vi "Stop Log and Sequence.vi"(4 "Log Config Name (CSVDataLog)":string="CSVDataLog", 5 "Session Complete Event Ref":T1, 6 "Sequence Name":string, 7 "Stim Stopped? (F)":bool=TRUE, 8 "error in (no error)":errorcluster, 10 "WorkspaceManager":T2, 11 "Stim Session":T3) -> (0 "error out":errorcluster, 1 "Pass?":bool, 2 "WorkspaceManager out":T2, 3 "Stim Session out":T3)   [LabVIEW 2011]
uses:
  <vilib>/NI Veristand/Execution/Workspace/WorkspaceAPI.ctl
  NationalInstruments.VeriStand.ClientAPI
  <vilib>/NI Veristand/Execution/SequenceExecutionInterface/Stimulus Profile Session Ref.ctl
  <vilib>/NI Veristand/Execution/SequenceExecutionInterface/Session Event Ref.ctl
  NationalInstruments.VeriStand.DataTypes
  <vilib>/NI Veristand/Execution/Workspace/NI_VS Workspace ExecutionAPI.lvlib
  <vilib>/NI Veristand/Execution/SequenceExecutionInterface/NI_VS Sequence Execution Interface.lvlib
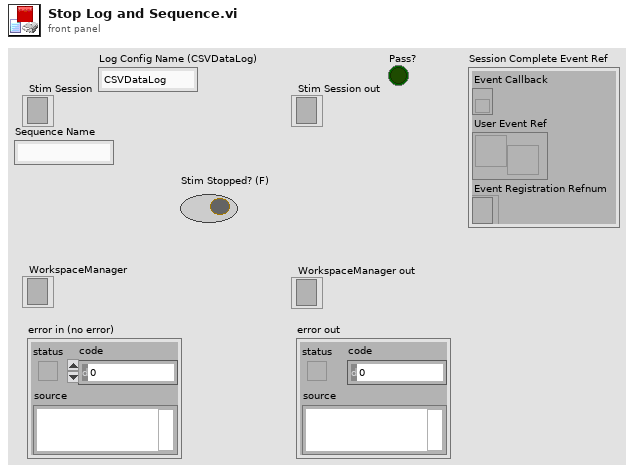
[diagram p1: front panel]
types:
  T1 = typedef "NI_VS Sequence Execution Interface.lvlib/Session Event Ref.ctl" = cluster{"Event Callback":refnum<k27>, "User Event Ref":refnum<user-event>, "Event Registration Refnum":refnum<event-registration>}
  T2 = typedef "NI_VS Workspace ExecutionAPI.lvlib/WorkspaceAPI.ctl" = refnum<k24>
  T3 = typedef "NI_VS Sequence Execution Interface.lvlib/Stimulus Profile Session Ref.ctl" = refnum<k24>
  T4 = typedef "NI_VS Sequence Execution Interface.lvlib/Data Value Ref.ctl" = refnum<k24>
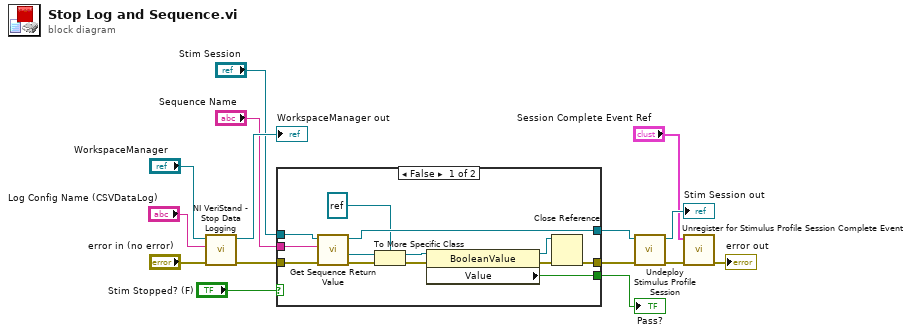
[diagram p0: block diagram]
diagram:
  n1 = call <vilib>:"NI VeriStand - Stop Data Logging.vi"("error in (no error)"="error in (no error)", "Data Log Configuration Name"="Log Config Name (CSVDataLog)", "WorkspaceManager in"="WorkspaceManager") -> ("error out"=w5:errorcluster, "WorkspaceManager out"=→"WorkspaceManager out":T2)  [unwired: 7 in]
  n2 = case shown="False" "Stim Stopped? (F)" {
    tunnel: "Sequence Name" -> [w28 _]
    tunnel: "Stim Session" -> [w27 w30]
    tunnel: [w26 w30] -> w6
    tunnel: w5 -> [w25 w29]
    tunnel: [w18 w29] -> w4
    tunnel: [w17 _] -> w3
    frame False {
      n3 = call <vilib>:"Get Sequence Return Value.vi"("error in (no error)"=w25, "Sequence Name"=w28, "Session Ref in"=w27) -> ("error out"=w24:errorcluster, "Data Value Ref"=w23:T4, "Session Ref out"=w26:T3)  [unwired: 5 in, 1 out]
      n4 = To More Specific Class(target class=refnum<k24> refnum ("reference"), reference=w23, error in=w24) -> (specific class reference=w22:refnum<k24>, error out=w21:errorcluster)
      n5 = property class="BooleanValue"(reference=w22, error in=w21) -> (reference out=w19:refnum<k24>, error out=w20:errorcluster, "Value"=w17:bool)
      n6 = Close Reference(reference=w19, error in (no error)=w20) -> (error out=w18:errorcluster)
    }
    frame True {
    }
  }
  "Pass?" <- w3
  n7 = call <vilib>:"Undeploy Stimulus Profile Session.vi"("error in (no error)"=w4, "Session Ref in"=w6) -> ("error out"=w11:errorcluster, "Session Ref out"=→"Stim Session out":T3)  [unwired: 8 in]
  n8 = call <vilib>:"Unregister for Stimulus Profile Session Complete Event.vi"("error in (no error)"=w11, "Session Complete Event Ref"="Session Complete Event Ref") -> ("error out"=→"error out":errorcluster)  [unwired: 9 in]
